vi "Write counter.vi"(8 "error in (no error)":errorcluster, 10 "Value":i32, 11 "Counter name (dflt=blank)":string) -> (0 "error out":errorcluster)   [LabVIEW 2021, in "Named Counters.lvlib"]
uses:
  Named Counters.lvlib
  Counter global variable.vi
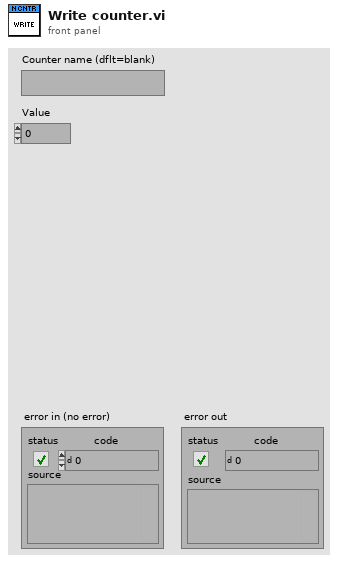
[diagram p1: front panel]
types:
  T1 = typedef "Named Counters.lvlib/Counter Cluster.ctl" = cluster{"Name":string, "Value":i32}
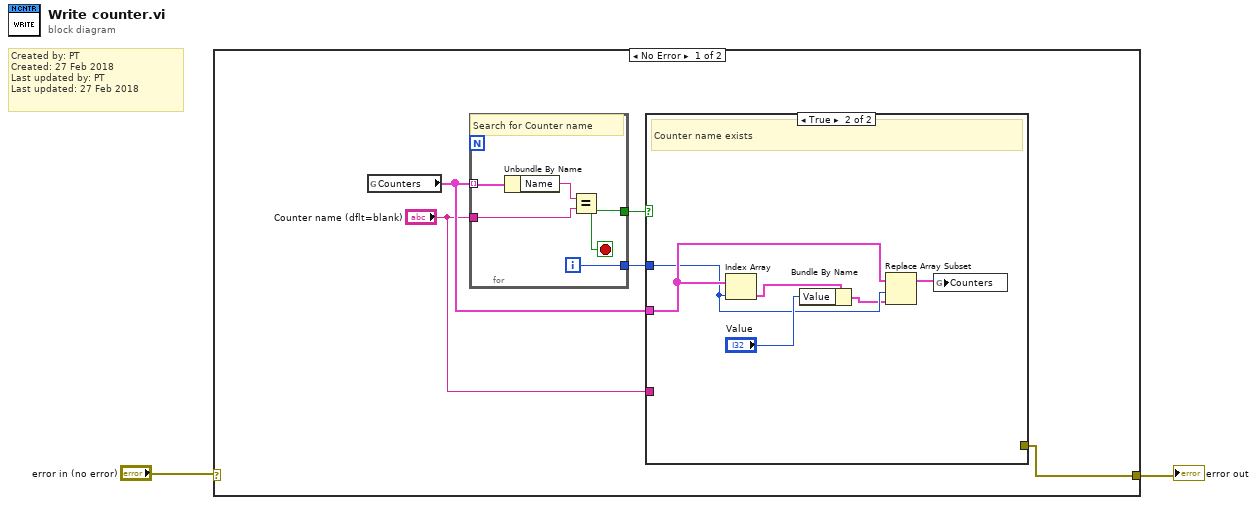
[diagram p0: block diagram]
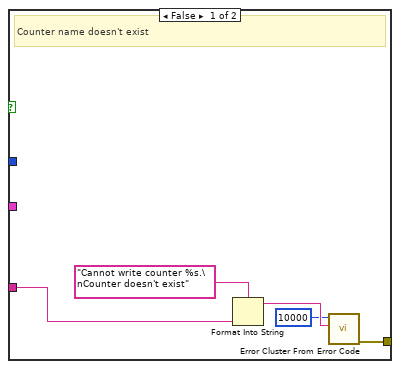
[diagram p2: hidden frame]
diagram:
  # "Created by: PT\nCreated: 27 Feb 2018\nLast updated by: PT\nLast updated: 27 Feb 2018"
  n1 = case shown="No Error" "error in (no error)" {
    selector: "error in (no error)" -> [_ w24]
    tunnel: [w3 w24] -> w1
    frame No Error {
      n2 = global read "Counter global variable.vi" "Counters"() -> (w6:T1[])
      n3 = for {
        tunnel: w6 -> [w23] mode=indexing
        tunnel: "Counter name (dflt=blank)" -> [w21]
        tunnel: [w20] -> w7
        tunnel: [w19] -> w4
        i -> [w19]
        stop <- w20 stop-if-true
        # "Search for Counter name"
        n4 = Unbundle By Name(w23) -> ("Name"=w22:string)
        n5 = Equal?(x=w22, y=w21) -> (x = y?=w20:bool)
      }
      n6 = case shown="True" w7 {
        tunnel: w6 -> [_ w16]
        tunnel: "Counter name (dflt=blank)" -> [w8 _]
        tunnel: w4 -> [_ w15]
        tunnel: [w9 _] -> w3
        frame False {
          # "Counter name doesn't exist"
          n7 = Format Into String(format string="Cannot write counter %s.\nCounter doesn't exist" ("error message (\"\")"), w8) -> (resulting string=w12:string)  [unwired: 2 in, 1 out]
          n8 = call <vilib>:"Error Cluster From Error Code.vi"("error message (\"\")"=w12, "error code (0)"=10000) -> ("error out"=w9:errorcluster)  [unwired: 7 in]
        }
        frame True {
          # "Counter name exists"
          n9 = Index Array(array=w16, index=w15) -> (element=w18:T1)
          n10 = Bundle By Name(cluster=w18, "Value"="Value") -> (w14:T1)
          n11 = Replace Array Subset(array=w16, new element=w14, index=w15) -> (w13:T1[])
          n12 = global write "Counter global variable.vi" "Counters"(w13) -> ()
        }
      }
    }
    frame Error {
    }
  }
  "error out" <- w1
